vi "Initialize Front Panel.vi"(8 "error in (no error)":errorcluster, 11 "Main ViewManager in":refnum<class "Main ViewManager.lvclass">) -> (0 "error out":errorcluster, 3 "Main ViewManager out":refnum<class "Main ViewManager.lvclass">)   [LabVIEW 2019, in "Main ViewManager.lvclass"]
doc: "<License>\nCopyright © 2017 Composed Systems, LLC | All rights reserved\nwww.composed.io\n\nAuthor: Ethan Stern <ethan.stern@composed.io>\n\nThis software is provided \"AS IS\" WITHOUT WARRANTIES, either express or implied, AND IS FOR EDUCATIONAL PURPOSES ONLY.\n</License>"
uses:
  <vilib>/gpm_packages/@cs/Car-wash/Source/Main ViewManager/Main ViewManager/Main ViewManager.lvclass
  <vilib>/gpm_packages/@cs/mva-viewable/Source/IViewManager/IViewManager/IViewManager.lvclass
  <vilib>/gpm_packages/@cs/mva-viewable/Source/IViewable/IViewable Messages/Insert Front Panel Msg/Insert Front Panel Msg.lvclass
  C:/Program Files/National Instruments/LabVIEW 2019/vi.lib/gpm_packages/@cs/mva-viewable/Source/IViewManager/IViewManager/IViewManager.lvclass
  C:/Program Files/National Instruments/LabVIEW 2019/vi.lib/gpm_packages/@cs/mva-viewable/Source/IViewable/IViewable/IViewable.lvclass
  C:/Program Files/National Instruments/LabVIEW 2019/vi.lib/gpm_packages/@cs/mva-viewable/Source/ActorEvents/IEventAggregator/IEventAggregator.lvclass
  C:/Program Files/National Instruments/LabVIEW 2019/vi.lib/gpm_packages/@cs/mva-core/Source/IObserver/IObserver/IObserver.lvclass
  C:/Program Files/National Instruments/LabVIEW 2019/vi.lib/ActorFramework/Actor/Actor.lvclass
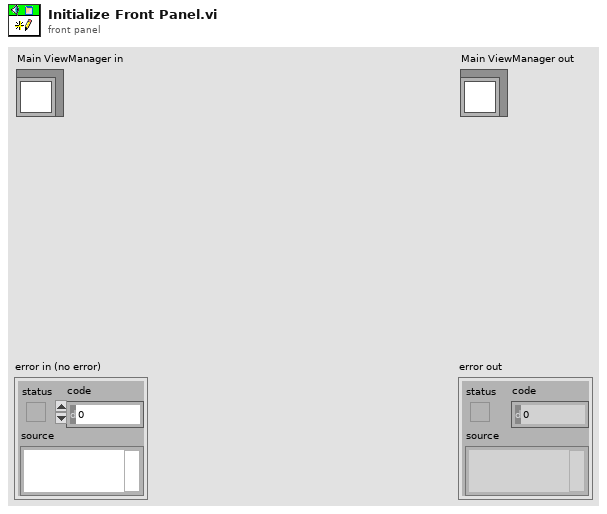
[diagram p1: front panel]
types:
  T1 = typedef "IViewable.lvlib/ProtectedSubpanel.lvclass/Protected Subpanel Reference.ctl" = refnum<data-value>
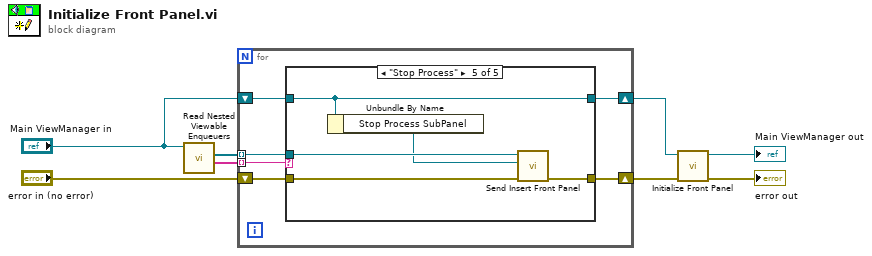
[diagram p0: block diagram]
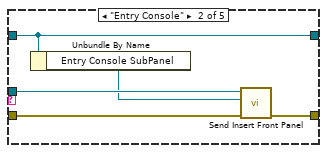
[diagram p3: hidden frame]
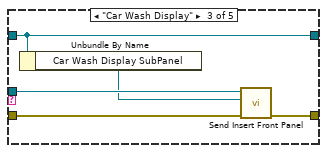
[diagram p4: hidden frame]
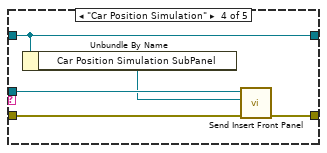
[diagram p5: hidden frame]
diagram:
  n1 = call <vilib>:"Read Nested Viewable Enqueuers.vi"("IViewManager in"="Main ViewManager in") -> ("Viewable Names"=w7:string[], "Nested Viewable Enqueuers"=w8:refnum<class "Message Enqueuer.lvclass">[])  [unwired: 9 in]
  n2 = for {
    tunnel: w8 -> [w12] mode=indexing
    tunnel: w7 -> [w9] mode=indexing
    shift-right: [w10] -> w1
    shift-left: "Main ViewManager in" -> [w11]
    shift-right: [w13] -> w4
    shift-left: "error in (no error)" -> [w14]
    n3 = case shown="\"Stop Process\"" w9 {
      tunnel: w14 -> [w15 w21 w26 w31 w36]
      tunnel: [w15 w20 w25 w30 w35] -> w13
      tunnel: w12 -> [_ w19 w24 w29 w34]
      tunnel: [w16 w18 w23 w28 w33] -> w10
      tunnel: w11 -> [w16 w18 w23 w28 w33]
      frame Default {
      }
      frame "Entry Console" {
        n4 = Unbundle By Name(w18) -> ("Entry Console SubPanel"=w17:T1)
        n5 = call <vilib>:"Send Insert Front Panel.vi"("error in (no error)"=w21, "Protected Subpanel"=w17, "Message Enqueuer"=w19) -> ("error out"=w20:errorcluster)  [unwired: 7 in, 1 out]
      }
      frame "Car Wash Display" {
        n6 = Unbundle By Name(w23) -> ("Car Wash Display SubPanel"=w22:T1)
        n7 = call <vilib>:"Send Insert Front Panel.vi"("error in (no error)"=w26, "Protected Subpanel"=w22, "Message Enqueuer"=w24) -> ("error out"=w25:errorcluster)  [unwired: 7 in, 1 out]
      }
      frame "Car Position Simulation" {
        n8 = Unbundle By Name(w28) -> ("Car Position Simulation SubPanel"=w27:T1)
        n9 = call <vilib>:"Send Insert Front Panel.vi"("error in (no error)"=w31, "Protected Subpanel"=w27, "Message Enqueuer"=w29) -> ("error out"=w30:errorcluster)  [unwired: 7 in, 1 out]
      }
      frame "Stop Process" {
        n10 = Unbundle By Name(w33) -> ("Stop Process SubPanel"=w32:T1)
        n11 = call <vilib>:"Send Insert Front Panel.vi"("error in (no error)"=w36, "Protected Subpanel"=w32, "Message Enqueuer"=w34) -> ("error out"=w35:errorcluster)  [unwired: 7 in, 1 out]
      }
    }
  }
  n12 = call-parent "Initialize Front Panel.vi"("error in (no error)"=w4, "IViewable in"=w1) -> ("error out"=→"error out":errorcluster, "IViewable out"=→"Main ViewManager out":refnum<class "Main ViewManager.lvclass">)  [unwired: 8 in]
